vi "hse-application_SetFpgaVersion.vi"(8 "error in":errorcluster, 11 "FPGA Version Number":string) -> (0 "error out":errorcluster)   [LabVIEW 2014, in "hse-application.lvclass"]
doc: "Stores the version number of the FPGA bitfile (if any) for later usage (display, logging, ...).\n\n\n\n____\nHAMPEL SOFTWARE ENGINEERING v0.12.0 (2018-09-13 18:21)"
uses:
  hse-application.lvclass
  hse-application.lvclass/hse-application.ctl
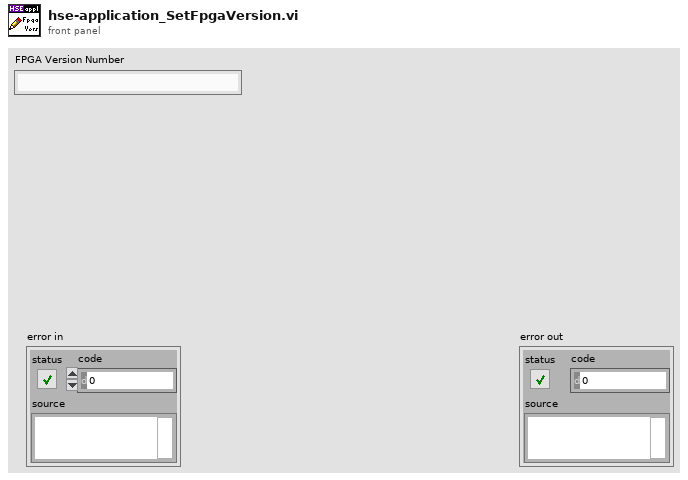
[diagram p1: front panel]
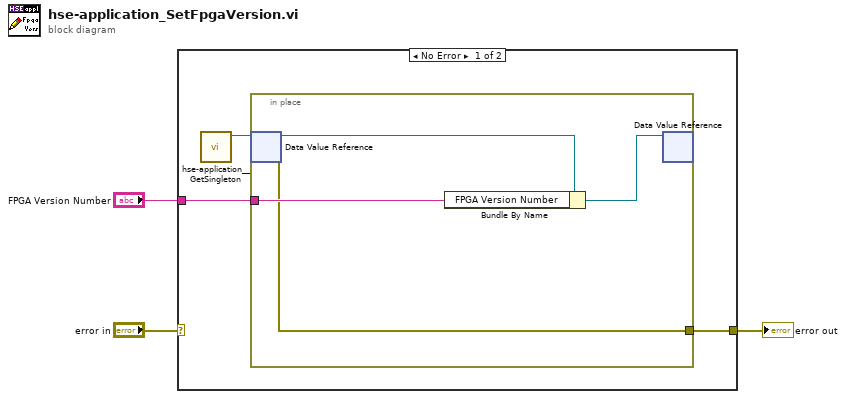
[diagram p0: block diagram]
diagram:
  n1 = case shown="No Error" "error in" {
    selector: "error in" -> [_ w11]
    tunnel: [w5 w11] -> w2
    tunnel: "FPGA Version Number" -> [w4 _]
    frame No Error {
      n2 = call "hse-application__GetSingleton.vi"() -> ("ApplicationClass DVR"=w6:refnum<data-value>)  [unwired: 10 in, 1 out]
      n3 = in-place {
        in-place-border: [w8] -> w5
        in-place-border: w4 -> [w9]
        n4 = in-place-dvr #1(w6) -> (w10:refnum<class "hse-application.lvclass">, w8:errorcluster)
        n5 = Bundle By Name(cluster=w10, "FPGA Version Number"=w9) -> (w7:refnum<class "hse-application.lvclass">)
        n6 = in-place-dvr #1(w7) -> ()  [unwired: 2 out]
      }
    }
    frame Error {
    }
  }
  "error out" <- w2
